vi "Generate Hardware Configuration File.vi"(8 "error in":errorcluster, 10 "hardware configuration file path":path, 11 "Ballard ARINC 429 custom device in":T1 format="%.0x") -> (0 "error out":errorcluster, 3 "Ballard ARINC 429 custom device out":T1 format="%.0x")   [LabVIEW 2020, in "Ballard ARINC 429 Scripting.lvlib"]
uses:
  Ballard ARINC 429 Scripting.lvlib
  Hardware Configuration/Ballard ARINC 429 Hardware Configuration.lvlib
  <vilib>/NI VeriStand/Custom Device API/Custom Device Item Ref.ctl
  <vilib>/NI VeriStand/Custom Device API/Custom Device API.lvlib
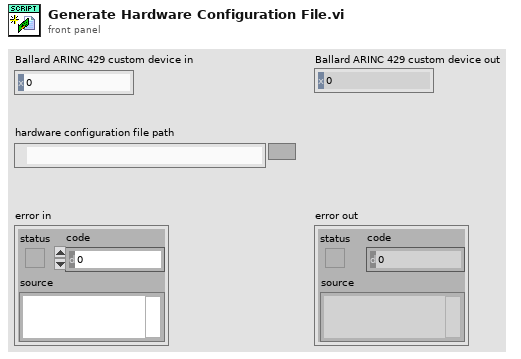
[diagram p1: front panel]
types:
  T1 = typedef "Custom Device API.lvlib/Custom Device Item Ref.ctl" = u64
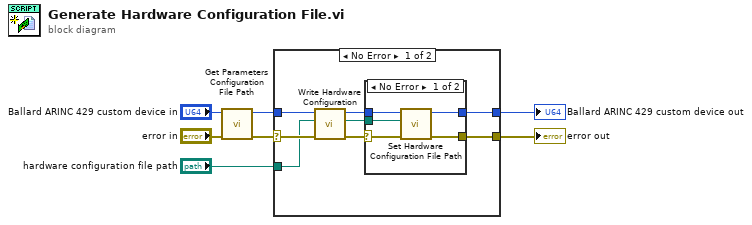
[diagram p0: block diagram]
diagram:
  n1 = call "Get Parameters Configuration File Path.vi"("error in"="error in", "Ballard ARINC 429 custom device in"="Ballard ARINC 429 custom device in") -> ("error out"=w5:errorcluster, "Ballard ARINC 429 custom device  out"=w4:T1)  [unwired: 6 in, 2 out]
  n2 = case shown="No Error" w5 {
    selector: w5 -> [w15 w23]
    tunnel: w4 -> [w14 w24]
    tunnel: "hardware configuration file path" -> [w13 _]
    tunnel: [w9 w23] -> w2
    tunnel: [w8 w24] -> w1
    frame No Error {
      n3 = call "Write Hardware Configuration.vi"("error in"=w15, "path"=w13, "custom device"=w14) -> ("error out"=w12:errorcluster, "path out"=w10:path, "custom device out"=w11:T1)  [unwired: 6 in]
      n4 = case shown="No Error" w12 {
        selector: w12 -> [w20 w22]
        tunnel: w11 -> [w19 w21]
        tunnel: w10 -> [w18 _]
        tunnel: [w17 w22] -> w9
        tunnel: [w16 w21] -> w8
        frame No Error {
          n5 = call "Set Hardware Configuration File Path.vi"("error in"=w20, "hardware configuration file path"=w18, "Ballard ARINC 429 custom device in"=w19) -> ("error out"=w17:errorcluster, "Ballard ARINC 429 custom device out"=w16:T1)  [unwired: 7 in]
        }
        frame Error {
        }
      }
    }
    frame Error {
    }
  }
  "error out" <- w2
  "Ballard ARINC 429 custom device out" <- w1
